vi "Get Public API.vi"(8 "error in (no error)":errorcluster, 11 "Instrument in":refnum<class "Instrument.lvclass">) -> (0 "error out":errorcluster, 2 "Commands":string[](array[string]), 3 "Instrument out":refnum<class "Instrument.lvclass">)   [LabVIEW 2016, in "Instrument.lvclass"]
uses:
  Instrument.lvclass
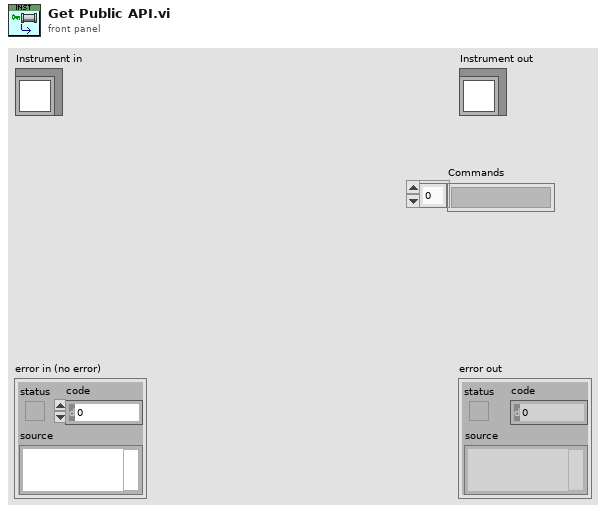
[diagram p1: front panel]
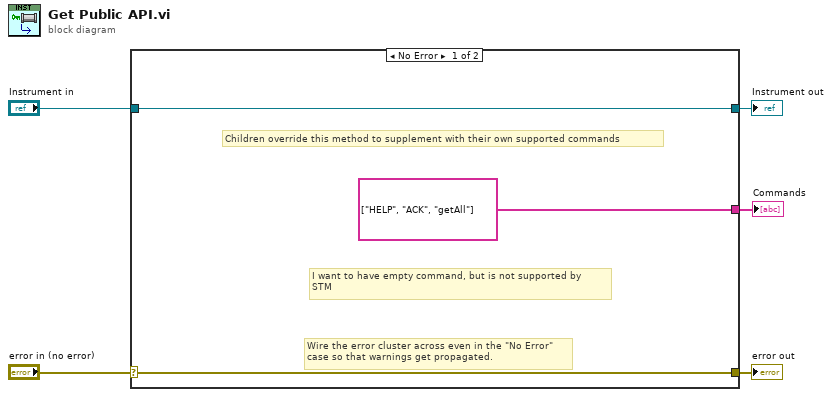
[diagram p0: block diagram]
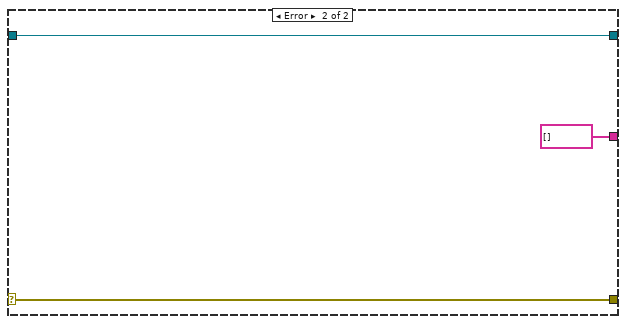
[diagram p2: hidden frame]
diagram:
  n1 = case shown="No Error" "error in (no error)" {
    selector: "error in (no error)" -> [w7 w11]
    tunnel: [w7 w11] -> w4
    tunnel: [w8 w10] -> w2
    tunnel: "Instrument in" -> [w8 w10]
    tunnel: [string[] ["HELP", "ACK", "getAll"] ("Array") string[] [] ("Array")] -> w1
    frame No Error {
      # "I want to have empty command, but is not supported by\nSTM"
      # "Children override this method to supplement with their own supported commands"
      # "Wire the error cluster across even in the \"No Error\"\ncase so that warnings get propagated."
    }
    frame Error {
    }
  }
  "error out" <- w4
  "Instrument out" <- w2
  "Commands" <- w1
